vi "Config VacuumLine.vi"(8 "error in (no error)":errorcluster, 11 "Configuration in":refnum<class "Configuration.lvclass">) -> (0 "error out":errorcluster, 3 "Configuration out":refnum<class "Configuration.lvclass">)   [LabVIEW 2016, in "Hardware.lvlib" / "VacuumLine.lvlib" / "VacuumLine Configuration.lvclass"]
uses:
  <userlib>/Common Components/Hardware/Abstract System/VacuumLine/VacuumLine Config/VacuumLine Configuration.lvclass
  <userlib>/Configuration Dialog Actor/Configuration.lvclass
  <userlib>/Common Components/Hardware/Abstract System/VacuumLine/VacuumLine/VacuumLine Params.ctl
  <userlib>/Common Components/Hardware/Abstract System/VacuumLine/VacuumLine/Valve Complex.ctl
  <userlib>/Common Components/Hardware/Abstract System/VacuumLine/VacuumLine/Logic Cluster.ctl
  C:/Program Files (x86)/National Instruments/LabVIEW 2016/user.lib/Configuration Dialog Actor/Configuration.lvclass
  C:/Program Files (x86)/National Instruments/LabVIEW 2016/vi.lib/ActorFramework/Actor/Actor.lvclass
  <userlib>/Common Components/Hardware/Abstract System/VacuumLine/VacuumLine Config/VacuumLine Configuration.lvclass/VacuumLine Configuration.ctl
  <userlib>/Common Components/Hardware/Abstract System/VacuumLine/VacuumLine/VacuumLine.lvclass/VacuumLine.ctl
  <vilib>/ActorFramework/Actor/Actor.lvclass/Actor.ctl
  <userlib>/Common Components/Hardware/Abstract System/VacuumLine/VacuumLine/Read VacuumLine Params.vi
  <userlib>/Common Components/Hardware/Abstract System/VacuumLine/VacuumLine/Write VacuumLine Params.vi
  <vilib>/ActorFramework/Actor/Actor.lvclass
  <userlib>/Common Components/Hardware/Abstract System/VacuumLine/VacuumLine/VacuumLine.lvclass
panel:
  in  "Position Params":T1 {"max( |Motor Pos - LRF Distance| )" min=0.0}
  in  "Revert":bool
  in  "Apply":bool
  # "Pin#"
  # "Location"
  # "Tolerance"
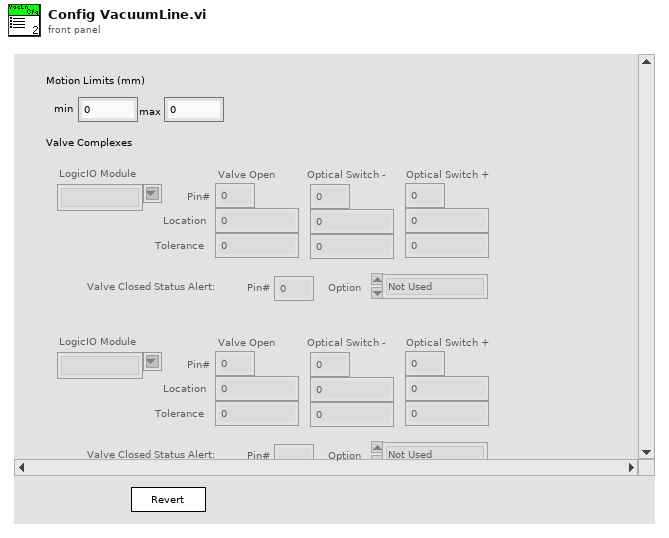
[diagram p1: front panel]
types:
  T1 = typedef "Hardware.lvlib/VacuumLine.lvlib/VacuumLine.lvclass/VacuumLine Params.ctl" = cluster{"Motion Limits":cluster{"min":dbl, "max":dbl}, "Valve Complexes":T2[], "max( |Motor Pos - LRF Distance| )":dbl}
  T2 = typedef "Hardware.lvlib/VacuumLine.lvlib/VacuumLine.lvclass/Valve Complex.ctl" = cluster{"LogicIO Module":string, "Valve Open":T3, "Optical Switch -":T3, "Optical Switch +":T3, "Valve Closed Status Alert":cluster{"Pin#":u8, "Option":enum16{"Not Used", "Normally Closed"}}}
  T3 = typedef "Hardware.lvlib/VacuumLine.lvlib/VacuumLine.lvclass/Logic Cluster.ctl" = cluster{"Pin#":u8, "Location":dbl, "Tolerance":dbl}
  T4 = cluster{"LogicIO Module":bool, "Valve Open":cluster{"Pin#":bool, "Location":bool, "Tolerance":bool}, "Optical Switch -":cluster{"Pin#":bool, "Location":bool, "Tolerance":bool}, "Optical Switch +":cluster{"Pin#":bool, "Location":bool, "Tolerance":bool}, "Valve Closed Status Alert":cluster{"Pin#":bool, "Option":bool}}[]
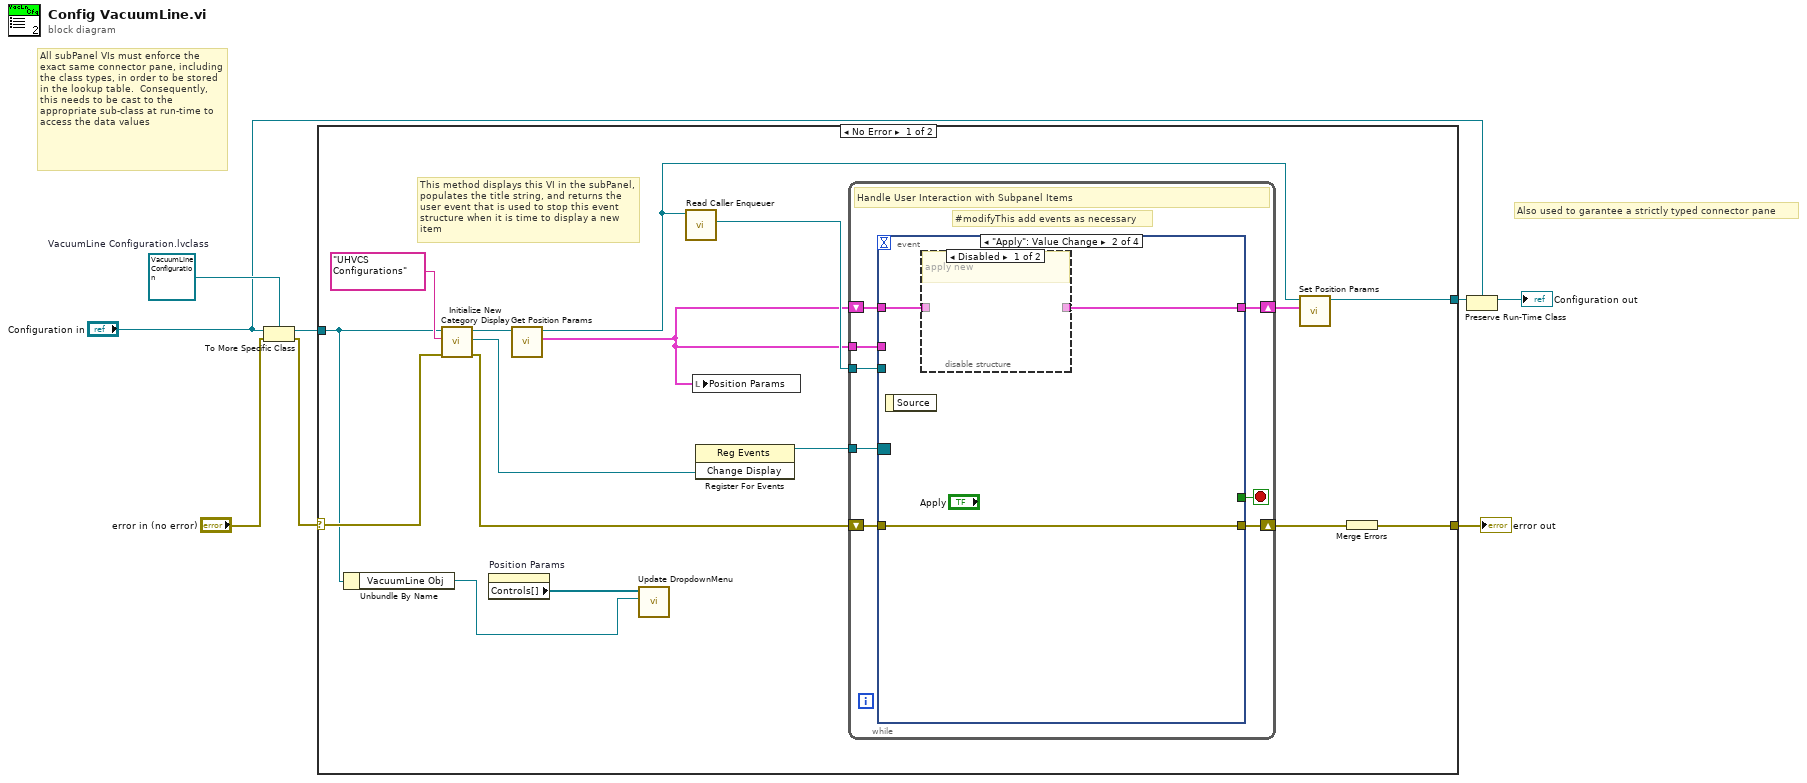
[diagram p0: block diagram]
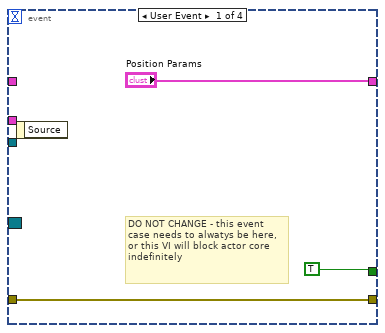
[diagram p2: hidden frame]
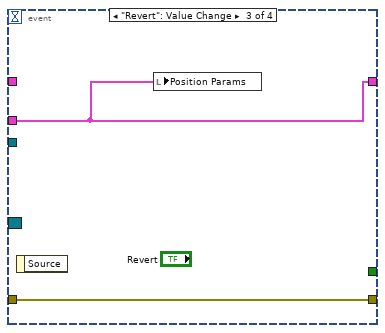
[diagram p4: hidden frame]
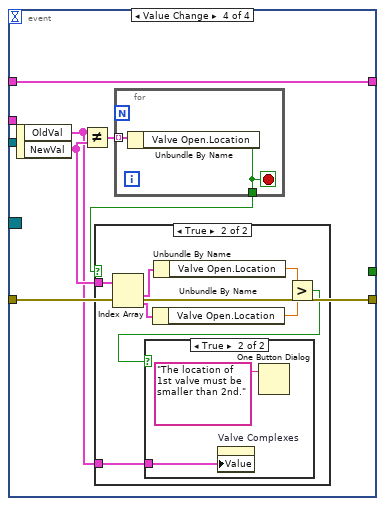
[diagram p5: hidden frame]
diagram:
  w5 = refnum<class "VacuumLine Configuration.lvclass"> refnum  # VacuumLine Configuration.lvclass
  # "Also used to garantee a strictly typed connector pane"
  # "All subPanel VIs must enforce the exact same connector pane, including the class types, in order to be stored in the lookup table.  Consequently, this needs to be cast to the appropriate sub-class at run-time to access the data values"
  n1 = To More Specific Class(target class=w5, reference="Configuration in", error in="error in (no error)") -> (specific class reference=w6:refnum<class "VacuumLine Configuration.lvclass">, error out=w1:errorcluster)
  n2 = case shown="No Error" w1 {
    selector: w1 -> [w18 w59]
    tunnel: w6 -> [w10 w60]
    tunnel: [w13 w60] -> w8
    tunnel: [w24 w59] -> w7
    frame No Error {
      # "This method displays this VI in the subPanel, populates the title string, and returns the user event that is used to stop this event structure when it is time to display a new item"
      n3 = Unbundle By Name(w10) -> ("VacuumLine Obj"=w9:refnum<class "VacuumLine.lvclass">)
      n4 = call <userlib>:"Initialize New Category Display.vi"("error in (no error)"=w18, "Name to Display"="UHVCS Configurations", "Configuration in"=w10) -> ("error out"=w19:errorcluster, "Change Display"=w22:refnum<user-event>, "Configuration Out"=w16:refnum<class "VacuumLine Configuration.lvclass">)  [unwired: 6 in]
      n5 = property on="Position Params" class="Clust (strict)"() -> ("Controls[]"=w11:refnum<vi>[])  [unwired: 2 in, 2 out]
      n6 = call <userlib>:"Get Position Params.vi"("VacuumLine Configuration in"=w16) -> ("Position Params"=w12:T1, "VacuumLine Configuration out"=w14:refnum<class "VacuumLine Configuration.lvclass">)  [unwired: 8 in, 1 out]
      n7 = call <userlib>:"Update DropdownMenu.vi"("VacuumLine Obj"=w9, "Controls[]"=w11) -> ()  [unwired: 10 in]
      n8 = call <vilib>:"Read Caller Enqueuer.vi"("Actor"=w14) -> ("Caller Enqueuer"=w17:refnum<class "Message Enqueuer.lvclass">)  [unwired: 10 in]
      n9 = local write "Position Params"(w12) -> ()
      n10 = register-events(w22) -> (reference out=w21:refnum<event-registration>)  [unwired: 2 in, 1 out]
      n11 = while {
        tunnel: w21 -> [w31]
        shift-right: [w30] -> w20
        shift-left: w19 -> [w29]
        shift-right: [w27] -> w15
        shift-left: w12 -> [w28]
        tunnel: w12 -> [w26]
        tunnel: w17 -> [w25]
        stop <- w32 stop-if-true
        # "#modifyThis add events as necessary"
        # "Handle User Interaction with Subpanel Items"
        n12 = event shown="[1] \"Apply\": Value Change" {
          selector: w31 -> [_ _ _ _]
          dyn-events: _ -> [_ _ _ _]
          timeout: _ -> [_ _ _ _]
          tunnel: [TRUE _ _ _] -> w32
          tunnel: [w35 w38 w41 w47] -> w30
          tunnel: w29 -> [w35 w38 w41 w47]
          tunnel: w28 -> [_ w36 _ w46]
          tunnel: ["Position Params" w37 w40 w46] -> w27
          tunnel: w26 -> [_ _ w40 _]
          tunnel: w25 -> [_ _ _ _]
          event User Event {
            # "DO NOT CHANGE - this event case needs to alwatys be here, or this VI will block actor core indefinitely"
            n13 = event-data() -> ()  [unwired: 1 in, 1 out]
          }
          event "Apply": Value Change {
            n14 = event-data() -> ()  [unwired: 1 in, 1 out]
            n15 = disable-structure shown="Disabled" {
              disable-tunnel: [_ w39] -> w37
              disable-tunnel: w36 -> [_ w39]
              frame Disabled {
                # "apply new"
              }
              frame Enabled {
              }
            }
          }
          event "Revert": Value Change {
            n16 = event-data() -> ()  [unwired: 1 in, 1 out]
            n17 = local write "Position Params"(w40) -> ()
          }
          event Value Change {
            n18 = event-data() -> ("OldVal"=w42:T2[], "NewVal"=w43:T2[])  [unwired: 1 in]
            n19 = Not Equal?(x=w42, y=w43) -> (x != y?=w45:T4)
            n20 = for {
              tunnel: w45 -> [w58] mode=indexing
              tunnel: [w57] -> w44
              stop <- w57 stop-if-true
              n21 = Unbundle By Name(w58) -> ("Valve Open.Location"=w57:bool)
            }
            n22 = case shown="True" w44 {
              tunnel: w43 -> [_ w49]
              tunnel: w42 -> [_ w48]
              frame False {
              }
              frame True {
                n23 = Index Array(array=w49) -> (element #1=w54:T2, element #2=w53:T2)  [unwired: 2 in]
                n24 = Unbundle By Name(w53) -> ("Valve Open.Location"=w51:dbl)
                n25 = Unbundle By Name(w54) -> ("Valve Open.Location"=w52:dbl)
                n26 = Greater?(x=w52, y=w51) -> (0:w50:bool)
                n27 = case shown="True" w50 {
                  tunnel: w48 -> [_ w55]
                  frame False {
                  }
                  frame True {
                    n28 = property on="Valve Complexes" class="Arr (strict)"("Value"=w55) -> ()  [unwired: 2 in, 2 out]
                    n29 = One Button Dialog(message="The location of 1st valve must be smaller than 2nd.") -> ()  [unwired: 1 in, 1 out]
                  }
                }
              }
            }
          }
        }
      }
      n30 = call <userlib>:"Set Position Params.vi"("Position Params"=w15, "VacuumLine Configuration in"=w14) -> ("VacuumLine Configuration out"=w13:refnum<class "VacuumLine Configuration.lvclass">)  [unwired: 8 in, 1 out]
      n31 = Merge Errors(w20) -> (w24:errorcluster)
    }
    frame Error {
    }
  }
  "error out" <- w7
  n32 = Preserve Run-Time Class(object in=w8, 2:"Configuration in") -> (object out=→"Configuration out":refnum<class "Configuration.lvclass">)  [unwired: 1 in, 1 out]
